vi "Check_Exp_Exists.vi"(8 "expId":string) -> (0 "expIndex":i32, 3 "exists":bool)   [LabVIEW 2019]
doc: "Checks if an experiment VI with the provided name exists and returns its index in case it does (or -1 if it doesn't)"
uses:
  Configuration/Global_Configurations.vi
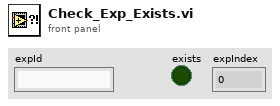
[diagram p1: front panel]
types:
  T1 = cluster{"Path":path, "Name":string, "Authors":string, "Keywords":string, "Description":string, "Cameras":cluster{"Base URL":string, "Path":string, "Name":string}[], "Sampling":cluster{"Sampled Variable":string, "Delta":dbl}[], "Sampling Freq":u32}[]
  T2 = cluster{"Path":path, "Name":string, "Authors":string, "Keywords":string, "Description":string, "Cameras":cluster{"Base URL":string, "Path":string, "Name":string}[], "Sampling":cluster{"Sampled Variable":string, "Delta":dbl}[], "Sampling Freq":u32}
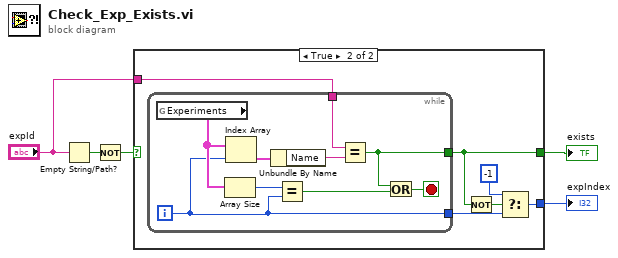
[diagram p0: block diagram]
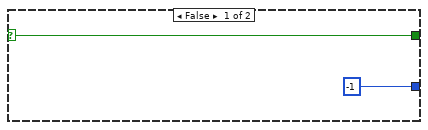
[diagram p2: hidden frame]
diagram:
  n1 = Empty String/Path?(string/path="expId") -> (empty?=w4:bool)
  n2 = Not(x=w4) -> (.not. x?=w3:bool)
  n3 = case shown="True" w3 {
    selector: w3 -> [w7 _]
    tunnel: [w7 w8] -> w5
    tunnel: "expId" -> [_ w13]
    tunnel: [-1 w11] -> w1
    frame False {
    }
    frame True {
      n4 = while {
        tunnel: w13 -> [w20]
        tunnel: [w16] -> w8
        tunnel: [w14] -> w10
        i -> [w14]
        stop <- w19 stop-if-true
        n5 = global read "Global_Configurations.vi" "Experiments"() -> (w18:T1)
        n6 = Array Size(array=w18) -> (size(s)=w17:i32)
        n7 = Index Array(array=w18, index=w14) -> (element=w22:T2)
        n8 = Unbundle By Name(w22) -> ("Name"=w21:string)
        n9 = Equal?(x=w17, y=w14) -> (x = y?=w15:bool)
        n10 = Equal?(x=w20, y=w21) -> (x = y?=w16:bool)
        n11 = Or(x=w16, y=w15) -> (x .or. y?=w19:bool)
      }
      n12 = Not(x=w8) -> (.not. x?=w9:bool)
      n13 = Select(t=-1, s=w9, f=w10) -> (s? t:f=w11:i32)
    }
  }
  "exists" <- w5
  "expIndex" <- w1
